vi "dboard eeprom set id.vi"(8 "error in (no error)":errorcluster, 10 "id":string, 11 "h":u64) -> (0 "error out":errorcluster, 3 "function return":u32(ring))   [LabVIEW 2023, in "uhd.lvlib"]
doc: "UHD_API uhd_error uhd_dboard_eeprom_set_id(uhd_dboard_eeprom_handle h, const char* id);"
uses:
  <userlib>/uhd/uhd.lvlib
  <userlib>/uhd/uhd.dll
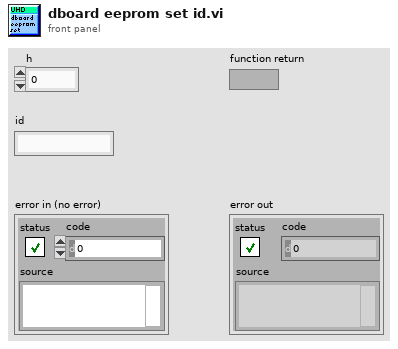
[diagram p1: front panel]
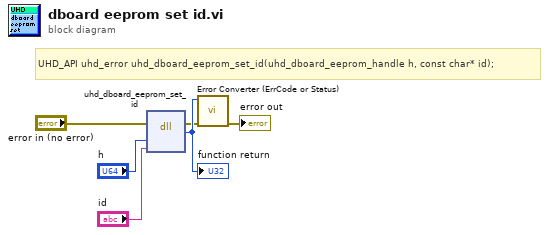
[diagram p0: block diagram]
diagram:
  # "UHD_API uhd_error uhd_dboard_eeprom_set_id(uhd_dboard_eeprom_handle h, const char* id);"
  n1 = dll-call lib="C:/Program Files/National Instruments/LabVIEW 2023/user.lib/uhd/uhd.*" fn="uhd_dboard_eeprom_set_id"(error in="error in (no error)", "h"="h", "id"="id") -> (error out=w2:errorcluster, w6:u32)  [unwired: 4 in, 1 out]
  "function return" <- w6
  n2 = call <userlib>:"Error Converter (ErrCode or Status).vi"("error in (no error)"=w2, "error code"=w6) -> ("error out"=→"error out":errorcluster)  [unwired: 9 in]
